vi "CRYMulti curves save.vi"(10 "Array of flattened data clusters":string[](array[string]), 11 "Datafile path":path) -> ()   [LabVIEW 2013]
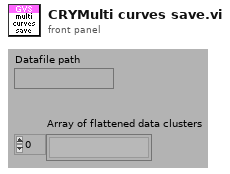
[diagram p1: front panel]
types:
  T1 = enum16{"open", "open or create", "create or replace", "create"}
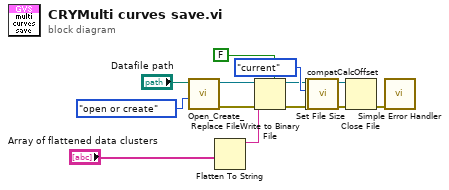
[diagram p0: block diagram]
diagram:
  n1 = call <vilib>:"Open_Create_Replace File.vi"("function (open:0)"=T1."open or create", "file path"="Datafile path") -> ("error out"=w8:errorcluster, "refnum"=w7:refnum<file>)  [unwired: 6 in, 2 out]
  n2 = Flatten To String(anything="Array of flattened data clusters") -> (data string=w6:string)  [unwired: 3 in, 2 out]
  n3 = Write to Binary File(file (use dialog)=w7, data=w6, error in=w8, 5:FALSE ("预置数组或字符串大小？(T)")) -> (refnum out=w10:refnum<file>, error out=w11:errorcluster)  [unwired: 2 in, 1 out]
  n4 = call <vilib>:"compatCalcOffset.vi"("error in"=w11, "pos mode (0:1)"=enum16{"start", "end", "current"}."current", "refnum"=w10) -> ("error out"=w3:errorcluster, "offset"=w2:i32, "dup refnum"=w1:refnum<file>)  [unwired: 6 in]
  n5 = Set File Size(4:w3, 6:w2, 7:w1) -> (0:w12:errorcluster, 3:w13:refnum<file>)
  n6 = Close File(refnum=w13, error in=w12) -> (error out=w9:errorcluster)  [unwired: 1 out]
  n7 = call <vilib>:"Simple Error Handler.vi"("error in (no error)"=w9) -> ()  [unwired: 4 in, 5 out]
